vi "Scanner OPC.vi"(8 "error in (no error)":errorcluster, 10 "OPC Notifier":refnum<notifier>, 11 "Hardware Resources in":T1={"Link"={"Connection"=enum."USB", "Host or IP address (TCP/IP)"="", "Port (Serial/USB)"="COM1"}, "VISA resource"="", "Writer Queue"=refnum, "Status"=FALSE}) -> (0 "error out":errorcluster, 3 "Hardware Resources out":T1={"Link"={"Connection"=enum."USB", "Host or IP address (TCP/IP)"="", "Port (Serial/USB)"="COM1"}, "VISA resource"="", "Writer Queue"=refnum, "Status"=FALSE})   [LabVIEW 2020, in "Hiden Scanner.lvlib"]
doc: "Generates sample waveforms according to the signal type in the HW Config input."
uses:
  Hiden Scanner.lvlib
  Scanner Hardware Configuration.ctl
  support/Message Queue/Message Cluster.ctl
  support/Message Queue/Message Queue.lvlib
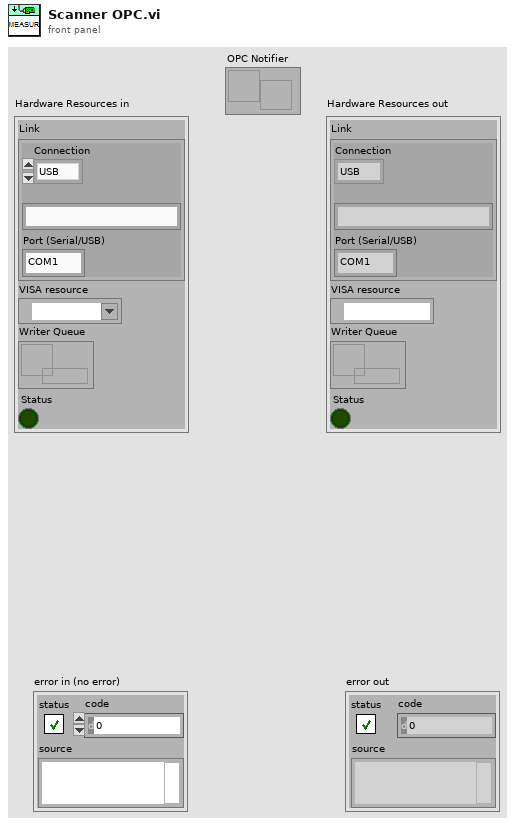
[diagram p1: front panel]
types:
  T1 = typedef "Hiden Scanner.lvlib/Scanner Hardware Configuration.ctl" = cluster{"Link":cluster{"Connection":enum16{"Serial", "TCP/IP", "USB"}, "Host or IP address (TCP/IP)":string, "Port (Serial/USB)":string}, "VISA resource":refnum<visa-resource-name>, "Writer Queue":refnum<queue>, "Status":bool}
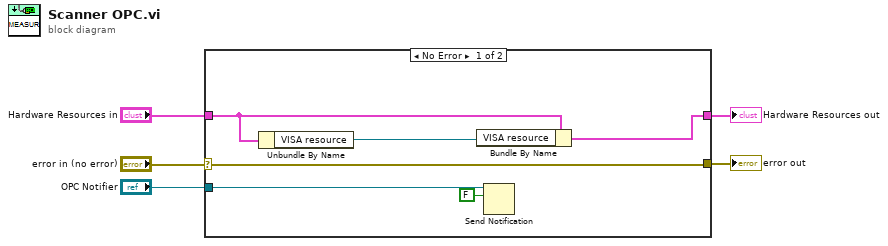
[diagram p0: block diagram]
diagram:
  n1 = case shown="No Error" "error in (no error)" {
    selector: "error in (no error)" -> [w8 w13]
    tunnel: [w8 w13] -> w4
    tunnel: "Hardware Resources in" -> [w11 w12]
    tunnel: [w10 w12] -> w2
    tunnel: "OPC Notifier" -> [w9 _]
    frame No Error {
      n2 = Unbundle By Name(w11) -> ("VISA resource"=w6:refnum<visa-resource-name>)
      n3 = Bundle By Name(cluster=w11, "VISA resource"=w6) -> (w10:T1)
      n4 = Send Notification(notification=FALSE, notifier=w9) -> ()  [unwired: 1 in, 2 out]
    }
    frame Error {
    }
  }
  "error out" <- w4
  "Hardware Resources out" <- w2
